vi "TH260_EnQError.vi"(8 "error in (no error)":errorcluster, 11 "Cmds_in":T1[](array[typedef])) -> (0 "error out":errorcluster, 3 "Cmds_out":T1[](array[typedef]))   [LabVIEW 2010]
uses:
  Types/TH260_UIThread_Cmds.ctl
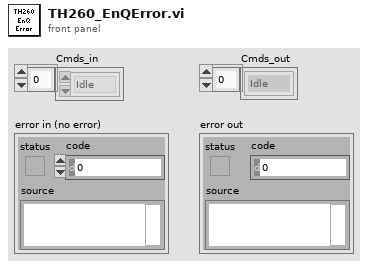
[diagram p1: front panel]
types:
  T1 = typedef "TH260_UIThread_Cmds.ctl" = enum16{"Idle", "Init", "SetInpChanEnable", "SetInpChanOffset", "SetInpChanCFD", "SetInpChanTrg", "SetInpChanDeadtime", "SetSyncDivider", "SetSyncCFD", "SetSyncTrg", "SetSyncOffset", "SetBinning", "SetHistoOffset", "SetHistoLen", "SetStopOvl", "SetBitShift", "SetHistoAcqTime", "GetRates", "StartMeas", "StopMeas", "AbortMeas", "GetResolution", "GetHisto", "ReadFiFo", "WriteStatus", "Resize", "EnableControls", "DisableControls", "Error", "Exit"}
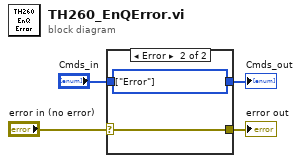
[diagram p0: block diagram]
diagram:
  n1 = case shown="Error" "error in (no error)" {
    selector: "error in (no error)" -> [_ w7]
    tunnel: [_ w7] -> w2
    tunnel: "Cmds_in" -> [w5 _]
    tunnel: [w5 w6] -> w4
    frame No Error {
    }
    frame Error {
      w6 = T1[] [enum."Error"] items=["Idle", "Init", "SetInpChanEnable", "SetInpChanOffset", "SetInpChanCFD", "SetInpChanTrg", "SetInpChanDeadtime", "SetSyncDivider", "SetSyncCFD", "SetSyncTrg", "SetSyncOffset", "SetBinning", "SetHistoOffset", "SetHistoLen", "SetStopOvl", "SetBitShift", "SetHistoAcqTime", "GetRates", "StartMeas", "StopMeas", "AbortMeas", "GetResolution", "GetHisto", "ReadFiFo", "WriteStatus", "Resize", "EnableControls", "DisableControls", "Error", "Exit"]
    }
  }
  "Cmds_out" <- w4
  "error out" <- w2
